vi "get_graph4report.vi"(8 "error in (no error)":errorcluster, 9 "D&T":string caption="Date and Time", 10 "ObjID":u16, 11 "connection reference":T1) -> (0 "error out":errorcluster, 2 "GraphArray":cluster{sgl, sgl, sgl[][]}[](array[cluster]), 3 "conn ref out":T1)   [LabVIEW 2010]
uses:
  <vilib>/addons/database/Connection.llb/Conn ObjectReference.ctl
  <vilib>/addons/database/NI_Database_API.lvlib
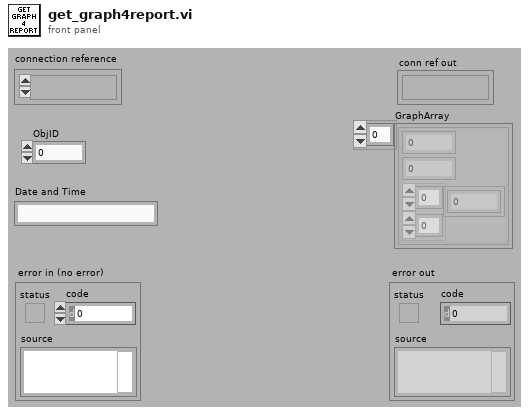
[diagram p1: front panel]
types:
  T1 = typedef "NI_Database_API.lvlib/Conn ObjectReference.ctl" = refnum<k1>
  T2 = cluster{"recordset data[0]":variant, "recordset data[1]":variant}
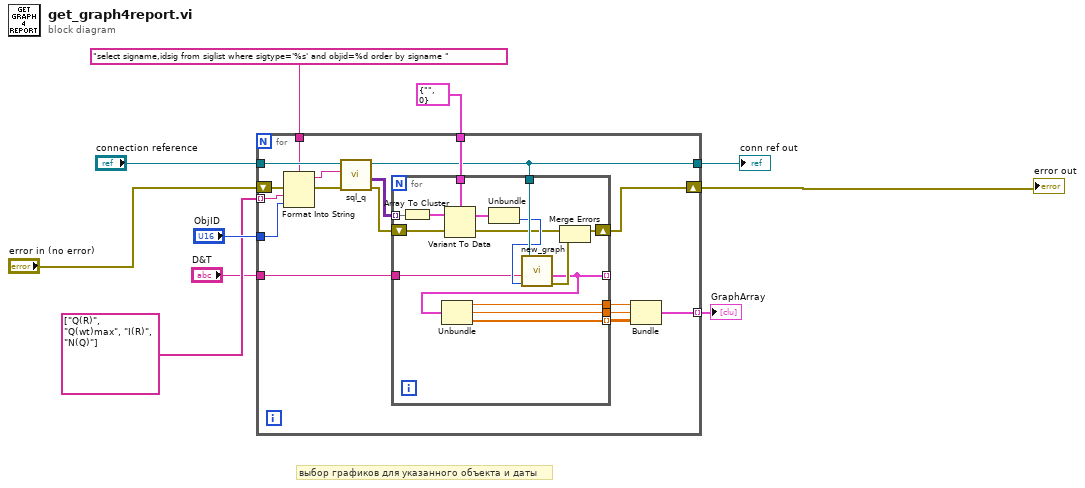
[diagram p0: block diagram]
diagram:
  # "выбор графиков для указанного объекта и даты"
  n1 = for {
    tunnel: [w16] -> w2
    tunnel: "connection reference" -> [w27]
    tunnel: cluster{string, i32} {"", 0} -> [w25]
    tunnel: "select signame,idsig from siglist where sigtype='%s' and objid=%d order by signame " ("SQL query") -> [w19]
    tunnel: "ObjID" -> [w18]
    shift-right: [w23] -> w3
    shift-left: "error in (no error)" -> [w21]
    tunnel: string[] ["Q(R)", "Q(wt)max", "I(R)", "N(Q)"] -> [w17] mode=indexing
    tunnel: "D&T" -> [w15]
    tunnel: [w11] -> w1 mode=indexing
    n2 = Format Into String(format string=w19, error in=w21, w17, w18) -> (resulting string=w20:string, error out=w22:errorcluster)  [unwired: 1 in]
    n3 = call "sql_q.vi"("error in"=w22, "SQL query"=w20, "connect ref"=w27) -> ("error out"=w24:errorcluster, "recordset data"=w26:variant[][], "conn ref out"=w16:T1)  [unwired: 1 in, 1 out]
    n4 = for {
      tunnel: w26 -> [w41] mode=indexing
      tunnel: w25 -> [w42]
      shift-right: [w32] -> w23
      shift-left: w24 -> [w39]
      tunnel: w16 -> [w36]
      tunnel: w15 -> [w34]
      tunnel: [w31] -> _ mode=indexing
      tunnel: [w30] -> w14
      tunnel: [w29] -> w13
      tunnel: [w28] -> w12 mode=indexing
      n5 = Array To Cluster(array=w41) -> (cluster=w40:T2)
      n6 = Variant To Data(error in=w39, Variant=w40, type=w42) -> (error out=w33:errorcluster, data=w38:cluster{string, i32})
      n7 = Unbundle(w38) -> (w35:i32)  [unwired: 1 out]
      n8 = call "new_graph.vi"("CurvesId"=w35, "D&T"=w34, "connection ref"=w36) -> ("error out"=w37:errorcluster, "Waveform Graph"=w31:cluster{sgl, sgl, sgl[]})  [unwired: 1 in, 2 out]
      n9 = Unbundle(w31) -> (w30:sgl, w29:sgl, w28:sgl[])
      n10 = Merge Errors(w33, w37) -> (w32:errorcluster)
    }
    n11 = Bundle(w14, w13, w12) -> (w11:cluster{sgl, sgl, sgl[][]})  [unwired: 1 in]
  }
  "error out" <- w3
  "conn ref out" <- w2
  "GraphArray" <- w1
